vi "FGV_ToProcessEvent.vi"(7 "Command":T1, 8 "error in (no error)":errorcluster) -> (0 "error out":errorcluster, 3 "ToProcessEvent":refnum<user-event>)   [LabVIEW 2011]
uses:
  EnumFgvEventCommand.ctl
  ToProcess.ctl
  ToProcess_EnumCommand.ctl
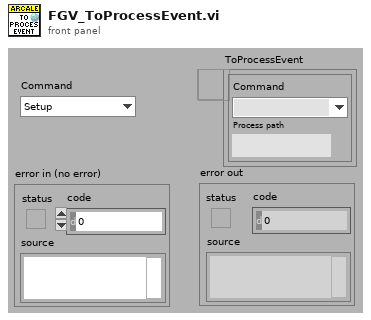
[diagram p1: front panel]
types:
  T1 = typedef "EnumFgvEventCommand.ctl" = enum16{"Setup", "Cleanup", "Get"}
  T2 = typedef "ToProcess.ctl" = cluster{"Command":T3, "Process path":path}
  T3 = typedef "ToProcess_EnumCommand.ctl" = enum16{"Show front panel", "Hide front panel"}
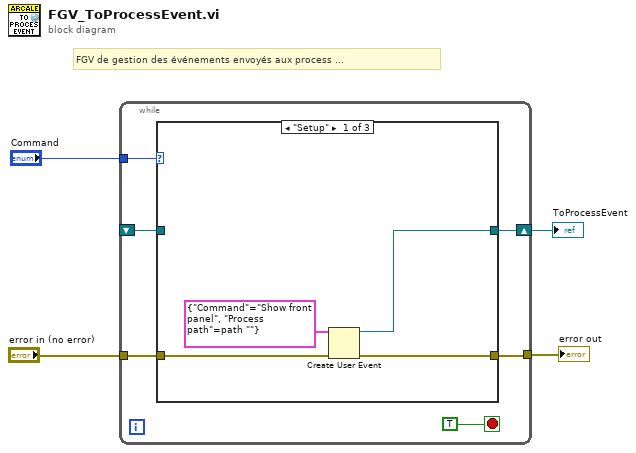
[diagram p0: block diagram]
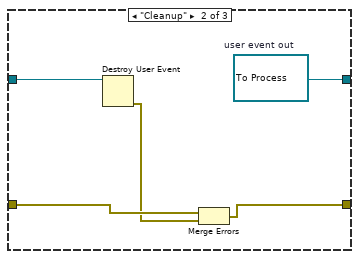
[diagram p2: hidden frame]
diagram:
  # "FGV de gestion des événements envoyés aux process ..."
  n1 = while {
    tunnel: "Command" -> [w9]
    tunnel: "error in (no error)" -> [w8]
    shift-right: [w7] -> w1
    shift-left: _ -> [w6]
    tunnel: [w5] -> w2
    stop <- TRUE stop-if-true
    n2 = case shown="\"Setup\"" w9 {
      tunnel: w8 -> [w14 w18 w20]
      tunnel: [w13 w15 w21] -> w7
      tunnel: w6 -> [_ w19 w21]
      tunnel: [w12 w16 w20] -> w5
      frame "Setup" {
        n3 = Create User Event(user event datatype=T2 {"Command"=enum."Show front panel", "Process path"=path ""} ("To Process"), error in=w14) -> (user event=w13:refnum<user-event>, error out=w12:errorcluster)
      }
      frame "Cleanup" {
        w15 = refnum<user-event> refnum  # user event out
        n4 = Destroy User Event(user event=w19) -> (error out=w17:errorcluster)  [unwired: 1 in]
        n5 = Merge Errors(w18, w17) -> (w16:errorcluster)
      }
      frame "Get" {
      }
    }
  }
  "error out" <- w2
  "ToProcessEvent" <- w1
